vi "Write_HTML_To_WebBrowser_ActiveX.vi"(8 "error in (no error)":errorcluster, 10 "stringHTML":string="<!DOCTYPE html PUBLIC \"-//W3C//DTD HTML 4.01 Transitional//EN\">\r\n<html>\r\n  <head>\r\n    <meta http-equiv=\"content-type\" content=\"text/html; charset=UTF-8\">\r\n    <title>main</title>\r\n  </head>\r\n  <body oncontextmenu=\"return false;\">\r\n    <h1><font color=\"#ff0000\"><b>CerberoII<font size=\"+3\"><sup>®</sup></font>\r\n          HELP</b></font></h1>\r\n    <div align=\"center\">\r\n      <div align=\"left\">\r\n        <h2 align=\"left\"><font color=\"#3333ff\">MAIN WINDOW</font><br>\r\n        </h2>\r\n        In this main window you can access all the CerberoII\r\n        funtionalities. You can directly change the main parameters,\r\n        monitor the analysis and see the results, get an overview of the\r\n        current system status and check the product informations. <br>\r\n        The following image shows an example of RSP (reference standard\r\n        pipe) inspection, where the main window parts have been\r\n        highlighted and described in this document.<br>\r\n        <br>\r\n      </div>\r\n      <div align=\"left\"><img src=\"main_window_plus_numbers.PNG\"\r\n          alt=\"main_window\" width=\"1501\" height=\"794\"></div>\r\n      <h2 align=\"left\">2D chart</h2>\r\n      <div align=\"left\">This chart is composed of three graps:<br>\r\n        <ul>\r\n          <li>2D intensity chart: it shows the inspection result in a\r\n            graph where on the X-axis there is the time, the Y-axis the\r\n            corresponding channel and the Z-axis corresponds to the\r\n            intensity of the signal in that point. The color scale at\r\n            the bottom of the chat shows the corresponding Z-value,\r\n            expressed in Volts;<br>\r\n          </li>\r\n          <li>max-min chart: it is above the 2D chart, and it represents\r\n            the maximum and the minimum value, expressed in Volts, of\r\n            all the signals for each sampling time. The yellow dashed\r\n            thresholds represent the current level of the pre-trigger;</li>\r\n          <li>max-min holder: placed at the right side of the 2D chart,\r\n            this graph holds the maximum and the minimum signal values\r\n            (in Volts) of the current inspection, reached by each\r\n            channel;</li>\r\n        </ul>\r\n        <p>It is possible to set the plot space, opening the <a\r\n            href=\"../system%20settings/system_settings.html\">settings\r\n            window</a> and changing the number of seconds to plot. <br>\r\n          At the end of the analysis the chart resizes to fill all the\r\n          available space. If the inspection last more than the\r\n          available number of seconds, the chart scroll until the end\r\n          inspection and doesn't resize.&nbsp; <br>\r\n          When the operating mode is 'auto' or 'semi-verification' the\r\n          charts automatically refreshes for every new inspection. In\r\n          all the other modes (for example 'manual') the chart behavior\r\n          is 'free running', and it resets when the data reach the end\r\n          of the plot. <br>\r\n          The element number 8 in the image above is the control palette\r\n          of the chart. At the end of the inspection you can use those\r\n          controls to operate on the graph. There are zoom, drag and\r\n          rescale options.<br>\r\n          By clicking directly on the 2D chart a tag appears, showing\r\n          the corresponding channel.<br>\r\n        </p>\r\n        <p>Placed to the right of the color scale there is the 'Clear'\r\n          button to manually clear all the charts.<br>\r\n        </p>\r\n        <h2 align=\"left\">Peak to peak chart</h2>\r\n        <p>This graph shows the maximum value peak to peak of the\r\n          signals in Volts. It includes the two thresholds: external '<b><font\r\n              color=\"#ffcc00\">EXT</font></b>' and internal '<b><font\r\n              color=\"#ff0000\">INT</font></b>'. They can be changed\r\n          directly from this graph, by dragging the corresponding line\r\n          on the graph or moving the letters of the sliding bar placed\r\n          to the right of the plot. The X-scale can be position\r\n          (expressed in meters) or time, depending on the line mode.<br>\r\n        </p>\r\n        When the system is in free running mode, it shows two plots:<br>\r\n        <ul>\r\n          <li>red plot: it represents the maximum peak to peak amplitude\r\n            of the channels you set as group 1 in the configuration\r\n            file;</li>\r\n          <li>light blue plot: it represents the maximum peak to peak\r\n            amplitude of the channels you set as group 2 in the\r\n            configuration file;</li>\r\n        </ul>\r\n        <p>During the inspection the chart shows only one white plot and\r\n          the X-axis is the position of the peak to peak value in\r\n          meters. If a defect is detected, a tag appears on the top of\r\n          it, indicating the type: <b>ED </b>for external defect and <b>ID\n\n\n\n\n\n\r\n          </b>when it's an internal one. In case the defect has both\r\n          internal and external components the tag will be ED. When the\r\n          inspection ends the chart automatically rescale the graph to\r\n          fill all the available space.<br>\r\n          The plot starts from the position you set as 'uninspected\r\n          head' (UH), and ends when the position of the data is equal to\r\n          the pipe length minus the 'uninspected tail' (UT) value. <br>\r\n          In case of points with position lower than the UH because of\r\n          the measurements uncertainty, that points will be plotted at\r\n          the UH position. On the other hand if the points have\r\n          positions greater than the pipe length minus UT, that points\r\n          will be forced at the pipe length minus UT position. <br>\r\n        </p>\r\n        <p>Placed at the bottom right of the chart there is the 'Clear'\r\n          button to manually clear the chart.<br>\r\n        </p>\r\n        <h2>Controls and indicators</h2>\r\n        <p>Referring to the picture above, the following numbered list\r\n          explains the meaning of the interface controls and indicators\r\n          and how to use them:<br>\r\n        </p>\r\n        <ol>\r\n          <li><b>Menu bar</b><b>: </b>contains four items (File, Tool,\r\n            System and '?') and allows you to manage all the\r\n            application.</li>\r\n          <ol>\r\n            <ul>\r\n              <li>File: under this item you can <b>load</b> a new\r\n                configuration, <b>save</b> the current configuration,\r\n                open the <a href=\"../wizard/wizard.html\"><u>wizard</u></a>\r\n                to create/modify a configuration, <b>close</b> the\r\n                application;</li>\r\n              <li>Tool: it allows you to make multiple things. Sorted by\r\n                item you can <b>Start/stop</b> the data stream, open\r\n                all the control windows (<a\r\n                  href=\"../calibration/calibration.html\"><u>Calibration</u></a>,\r\n                <a href=\"../criteria/criteria_window.html\"><u>Criteria</u></a>,\r\n                <a href=\"../vumeter/vumeter.html\"> <u>Vumeter</u></a>,\r\n                <a href=\"../stripchart%20Vpp/stripchart.html\"> <u>Stripchart-Vpp</u></a>,\r\n                <a href=\"../channels%20setting/channel_setting.html\"><u>Channel\n\n\n\n\n\n\r\n                    settings</u></a>,<u> <a\r\n                    href=\"../oscilloscope/oscilloscope.html\">Oscilloscope</a></u>,\r\n                <a href=\"../filters/filters.html\"><u>Filter</u></a>,<u>\r\n                  <a href=\"../create%20delta/create_deltas.html\"> Create\r\n                    delta</a></u>, <a\r\n                  href=\"../record%20data/record_data_window.html\"><u>Record\n\n\n\n\n\r\n                    data</u></a>), <b>update offset</b><b> </b>and <b>remove\n\n\n\n\n\r\n                  offset </b>of the data;</li>\r\n              <li>System: under this item you can find the <a\r\n                  href=\"../alarms/alarms.html\"><u>alarms</u></a> window\r\n                to monitor the alarms, the <a\r\n                  href=\"../live%20view/live_view.html\"><u>'live view'</u></a>\r\n                to check the raw data stream, the <a\r\n                  href=\"../system%20info/system_info.html\"><u>info</u></a>\r\n                window that shows all the system information, and the <a\r\n                  href=\"../system%20settings/system_settings.html\"><u>settings</u></a>\r\n                window where it's possible to change a lot of inspection\r\n                parameters;</li>\r\n              <li>'?': it shows the CerberoII software informations as\r\n                the version and the release date; <br>\r\n              </li>\r\n            </ul>\r\n          </ol>\r\n        </ol>\r\n        <ol>\r\n          <ol>\r\n            <ul>\r\n            </ul>\r\n          </ol>\r\n          <li><b>Shortcut buttons: </b>with these buttons you can\r\n            quickly access the main control windows</li>\r\n        </ol>\r\n        <table width=\"60%\" cellspacing=\"2\" cellpadding=\"2\" border=\"1\">\r\n          <tbody>\r\n            <tr>\r\n              <td valign=\"top\" align=\"center\"><img\r\n                  src=\"calib_button.PNG\" alt=\"calib_button\" width=\"51\"\r\n                  height=\"53\"><br>\r\n              </td>\r\n              <td valign=\"middle\" align=\"left\"><a\r\n                  href=\"../calibration/calibration.html\"><u>Calibration</u></a>:\r\n                to start the automatic equalization or calibration\r\n                process;</td>\r\n            </tr>\r\n            <tr>\r\n              <td valign=\"top\" align=\"center\"><img\r\n                  src=\"criteria_button.PNG\" alt=\"criteria_button\"\r\n                  width=\"51\" height=\"51\"></td>\r\n              <td valign=\"middle\" align=\"left\"><a\r\n                  href=\"../criteria/criteria_window.html\"><u>Criteria</u></a>:\r\n                to set the criteria parameters of the defects detection;</td>\r\n            </tr>\r\n            <tr>\r\n              <td valign=\"top\" align=\"center\"><img\r\n                  src=\"vumeter_button.PNG\" alt=\"vumeter_button\"\r\n                  width=\"53\" height=\"53\"><br>\r\n              </td>\r\n              <td valign=\"middle\" align=\"left\"><a\r\n                  href=\"../vumeter/vumeter.html\"><u>Vumeter</u></a>: to\r\n                manage all the channels gains;</td>\r\n            </tr>\r\n            <tr>\r\n              <td valign=\"top\" align=\"center\"><img\r\n                  src=\"stripchart_button.PNG\" alt=\"stripchart_button\"\r\n                  width=\"53\" height=\"52\"><br>\r\n              </td>\r\n              <td valign=\"middle\" align=\"left\"><a\r\n                  href=\"../stripchart%20Vpp/stripchart.html\"><u>Stripchart-Vpp</u></a>\r\n                (when it is not set as 'always visible' in the main\r\n                window): to see the peak to peak chart, the product\r\n                infomation and change the thresholds;</td>\r\n            </tr>\r\n            <tr>\r\n              <td valign=\"top\" align=\"center\"><img\r\n                  src=\"filter_button.PNG\" alt=\"filter_button\" width=\"53\"\r\n                  height=\"52\"><br>\r\n              </td>\r\n              <td valign=\"middle\" align=\"left\"><a\r\n                  href=\"../filters/filters.html\"><u>Filter</u></a>: to\r\n                set a lot of different types of filters;</td>\r\n            </tr>\r\n            <tr>\r\n              <td valign=\"top\" align=\"center\"><img\r\n                  src=\"oscilloscope_button.PNG\"\r\n                  alt=\"oscilloscope_button\" width=\"52\" height=\"53\"><br>\r\n              </td>\r\n              <td valign=\"middle\" align=\"left\"><a\r\n                  href=\"../oscilloscope/oscilloscope.html\"><u>Oscilloscope</u></a>:\r\n                to analyze the signals with a standard digital\r\n                oscolloscope;</td>\r\n            </tr>\r\n            <tr>\r\n              <td valign=\"top\" align=\"center\"><img src=\"save_button.PNG\"\r\n                  alt=\"save_button\" width=\"105\" height=\"35\"><br>\r\n              </td>\r\n              <td valign=\"middle\" align=\"left\"><u>Save config</u>: to\r\n                quickly save id/od configurations or a new one;</td>\r\n            </tr>\r\n            <tr>\r\n              <td valign=\"top\" align=\"center\"><img src=\"load_button.PNG\"\r\n                  alt=\"load_button\" width=\"106\" height=\"36\"><br>\r\n              </td>\r\n              <td valign=\"middle\" align=\"left\"><u>Load config</u>: to\r\n                quickly switch between id and od configurations (only\r\n                for similar configurations);</td>\r\n            </tr>\r\n            <tr>\r\n              <td valign=\"top\" align=\"center\"><img\r\n                  src=\"v_div_control.PNG\" alt=\"v_div_control\"\r\n                  width=\"110\" height=\"27\"><br>\r\n              </td>\r\n              <td valign=\"middle\" align=\"left\"><u>V/div control</u>: it\r\n                changes the scale of all the charts;</td>\r\n            </tr>\r\n          </tbody>\r\n        </table>\r\n        <ol>\r\n          <ol>\r\n            <ul>\r\n            </ul>\r\n          </ol>\r\n        </ol>\r\n        <ol start=\"3\">\r\n          <ol>\r\n            <ul>\r\n            </ul>\r\n          </ol>\r\n          <li><b>Thresholds and discrimination frequency: </b>using\r\n            this three controls you can set the two thresholds and the\r\n            discrimination frequency used for defects detection.</li>\r\n        </ol>\r\n        <table width=\"30%\" cellspacing=\"2\" cellpadding=\"2\" border=\"1\">\r\n          <tbody>\r\n            <tr>\r\n              <td valign=\"middle\" align=\"center\"><img\r\n                  src=\"ext_control.PNG\" alt=\"ext_control\" width=\"158\"\r\n                  height=\"36\"><br>\r\n              </td>\r\n              <td valign=\"middle\">External threshold control<br>\r\n              </td>\r\n            </tr>\r\n            <tr>\r\n              <td valign=\"top\" align=\"center\"><img src=\"int_control.PNG\"\r\n                  alt=\"int_threshold\" width=\"153\" height=\"33\"><br>\r\n              </td>\r\n              <td valign=\"middle\">Internal threshold control</td>\r\n            </tr>\r\n            <tr>\r\n              <td valign=\"top\" align=\"center\"><img\r\n                  src=\"discr_freq_control.PNG\"\r\n                  alt=\"discrimination_frequancy_control\" width=\"154\"\r\n                  height=\"34\"><br>\r\n              </td>\r\n              <td valign=\"middle\">Discrimination frequency control<br>\r\n              </td>\r\n            </tr>\r\n          </tbody>\r\n        </table>\r\n        <ol start=\"4\">\r\n          <li><b>Product informations: </b>they show the pipe number\r\n            under inspection, the batch name, the diameter, the\r\n            thickness, the pipe speed, the last plotted position and the\r\n            rotational speed in the case of rotating equipment;</li>\r\n        </ol>\r\n        <blockquote> <img src=\"product_info.PNG\" alt=\"product_info\"\r\n            width=\"238\" height=\"238\"><br>\r\n        </blockquote>\r\n        <ol start=\"5\">\r\n          <li><b>Status leds: </b>they give you a quick overview of the\r\n            actual situation.</li>\r\n        </ol>\r\n        <blockquote> <img src=\"leds.PNG\" alt=\"leds\" width=\"452\"\r\n            height=\"39\"><br>\r\n        </blockquote>\r\n        <ol start=\"6\">\r\n          <ol>\r\n            <ul>\r\n            </ul>\r\n          </ol>\r\n          <ul type=\"square\">\r\n            <li>Back-end: if on (green colour), the back-end application\r\n              is connected;</li>\r\n            <li>Pyxis: it indicates if the Pyxis device is connected or\r\n              not;</li>\r\n            <li>Level-1: when it is green the CerberoII is connected to\r\n              the PLC of the line;</li>\r\n            <li>Level-2: if green it means that the level-2 computer is\r\n              connected to the server created by the CerberoII;</li>\r\n            <li>Alarms: it can be red or green. If red, there is one or\r\n              more alarms active, otherwise it's green;</li>\r\n          </ul>\r\n          <ol>\r\n            <ul>\r\n            </ul>\r\n          </ol>\r\n        </ol>\r\n        <ol start=\"6\">\r\n          <ol>\r\n            <ul>\r\n            </ul>\r\n          </ol>\r\n          <li><b>System indicators:</b> these three indicators show the<i>\r\n            </i><i>line mode</i>, the CerberoII <i>status</i> and the\r\n            selected configuration;</li>\r\n        </ol>\r\n        <blockquote> <img src=\"system_indicators.PNG\"\r\n            alt=\"system_indicators\" width=\"826\" height=\"38\"><br>\r\n        </blockquote>\r\n        <ol start=\"7\">\r\n          <li><a\r\n              href=\"../last%20defect%20window/last_defect_window.html\"><u><b>Last\n\n\n\r\n                  defect window</b></u></a>: this button turns yellow\r\n            when a defect has been detected. When you click on it, you\r\n            open a window with all the defect\r\n            informations;&nbsp;&nbsp;&nbsp;</li>\r\n        </ol>\r\n        <blockquote> <b><img src=\"defect_led_off.PNG\"\r\n              alt=\"defect_led_off\" width=\"102\" height=\"81\">&nbsp;</b><b>\r\n            <font size=\"+3\">→</font></b><b><font size=\"+3\"> </font><img\r\n              src=\"defect_led_on.PNG\" alt=\"defect_led_on\" width=\"96\"\r\n              height=\"79\"></b><br>\r\n          <b> </b> </blockquote>\r\n        <ol start=\"8\">\r\n          <li><b>2D chart controls: </b>these buttons allows to operate\r\n            on the 2D chart; <br>\r\n          </li>\r\n        </ol>\r\n      </div>\r\n    </div>\r\n  </body>\r\n</html>\r\n", 11 "object in":refnum<class "WebBrowser_Mgmt.lvclass">) -> (0 "error out":errorcluster, 3 "object out":refnum<class "WebBrowser_Mgmt.lvclass">)   [LabVIEW 2016, in "WebBrowser_Mgmt.lvclass"]
uses:
  WebBrowser_Mgmt.lvclass
  Crypter/Crypter.lvclass
  WebBrowser_Mgmt.lvclass/WebBrowser_Mgmt.ctl
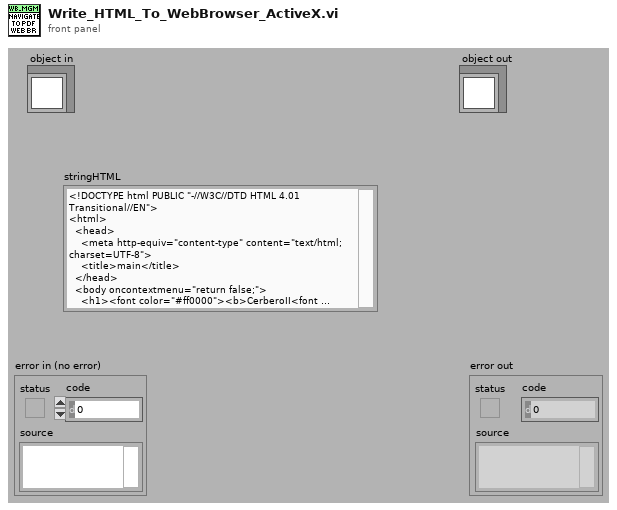
[diagram p1: front panel]
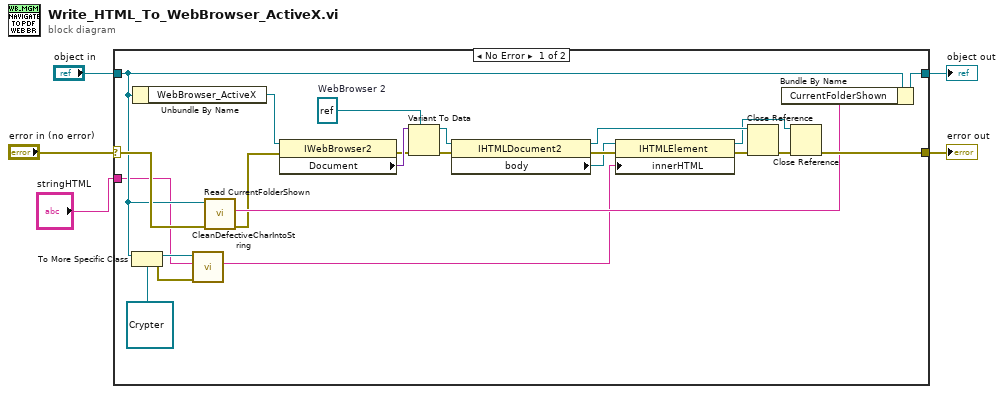
[diagram p0: block diagram]
diagram:
  n1 = case shown="No Error" "error in (no error)" {
    selector: "error in (no error)" -> [w16 w30]
    tunnel: [w24 w30] -> w4
    tunnel: [w18 w29] -> w2
    tunnel: "object in" -> [w12 w29]
    tunnel: "stringHTML" -> [w9 _]
    frame No Error {
      w23 = refnum<k7> refnum  # WebBrowser 2
      n2 = To More Specific Class(target class=refnum<class "Crypter.lvclass"> refnum ("object in"), reference=w12) -> (specific class reference=w10:refnum<class "Crypter.lvclass">, error out=w13:errorcluster)  [unwired: 1 in]
      n3 = Unbundle By Name(w12) -> ("WebBrowser_ActiveX"=w14:refnum<k7>)
      n4 = call-dynamic "CleanDefectiveCharIntoString.vi"("error in (no error)"=w13, "String In"=w9, "object in"=w10) -> ("String Out"=w8:string)  [unwired: 6 in, 2 out]
      n5 = call "Read CurrentFolderShown.vi"("error in (no error)"=w16, "WebBrowser_Mgmt in"=w12) -> ("error out"=w15:errorcluster, "CurrentFolderShown"=w17:string)  [unwired: 7 in, 1 out]
      n6 = property class="IWebBrowser2"(reference=w14, error in=w15) -> (error out=w19:errorcluster, "Document"=w21:variant)  [unwired: 1 out]
      n7 = Variant To Data(error in=w19, type=w23, Variant=w21) -> (data=w22:refnum<k7>, error out=w20:errorcluster)
      n8 = property class="IHTMLDocument2"(reference=w22, error in=w20) -> (reference out=w27:refnum<k7>, error out=w28:errorcluster, "body"=w6:refnum<k7>)
      n9 = property class="IHTMLElement"(reference=w6, error in=w28, "innerHTML"=w8) -> (reference out=w7:refnum<k7>, error out=w26:errorcluster)
      n10 = Close Reference(reference=w27, error in (no error)=w26) -> (error out=w25:errorcluster)
      n11 = Bundle By Name(cluster=w12, "CurrentFolderShown"=w17) -> (w18:refnum<class "WebBrowser_Mgmt.lvclass">)
      n12 = Close Reference(reference=w7, error in (no error)=w25) -> (error out=w24:errorcluster)
    }
    frame Error {
    }
  }
  "error out" <- w4
  "object out" <- w2
